vi "GOOP PROBE.vi"(11 "Probed Object":refnum<class>) -> (2 "Value String":string, 3 "Boolean":bool)   [LabVIEW 2019, in "GOOP Probe.lvlib"]
uses:
  GOOP Probe/GOOP Probe.lvlib
panel:
  out "Class Name":string
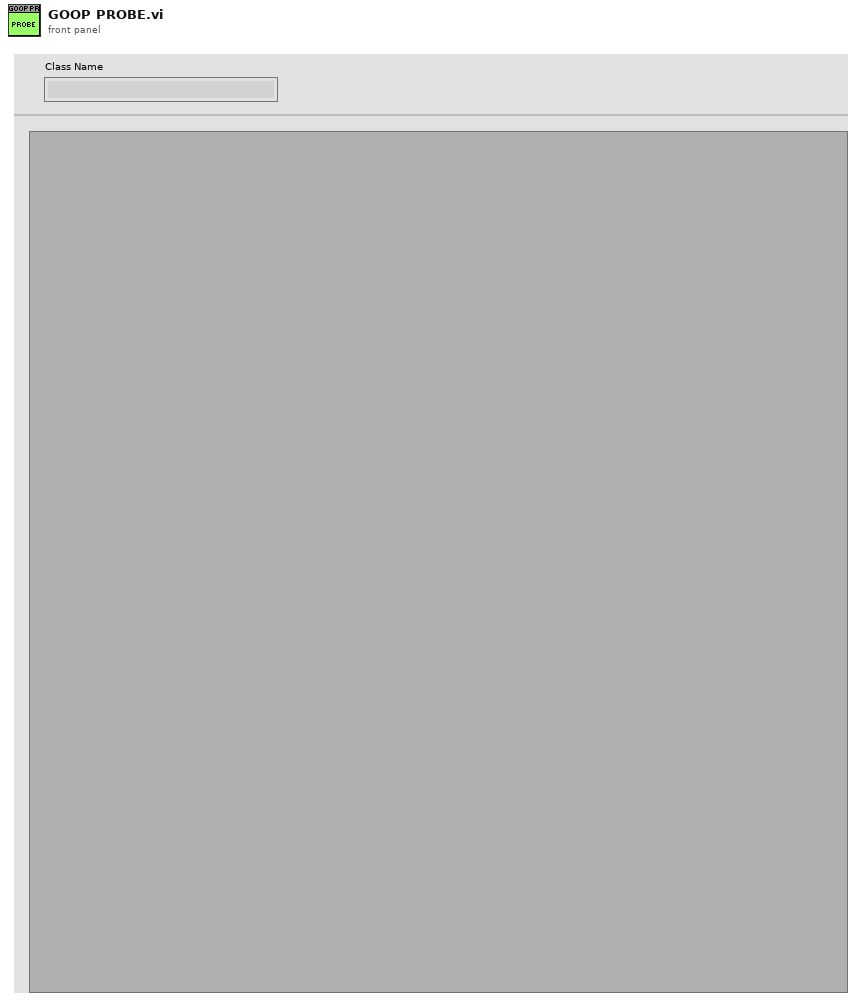
[diagram p1: front panel]
types:
  T1 = cluster{"Base Folder":path, "Cache Folder":path, "Cached Probe VI":path}
  T2 = cluster{"Object":refnum<class>, "FQN":string, "Class Name":string}
  T3 = typedef "GOOP Probe.lvlib/Level Data.ctl" = cluster{"Refnum":i32, "FQN":string, "Class Name":string, "ObjAtt.ctl Path":path, "Type":refnum<class>}
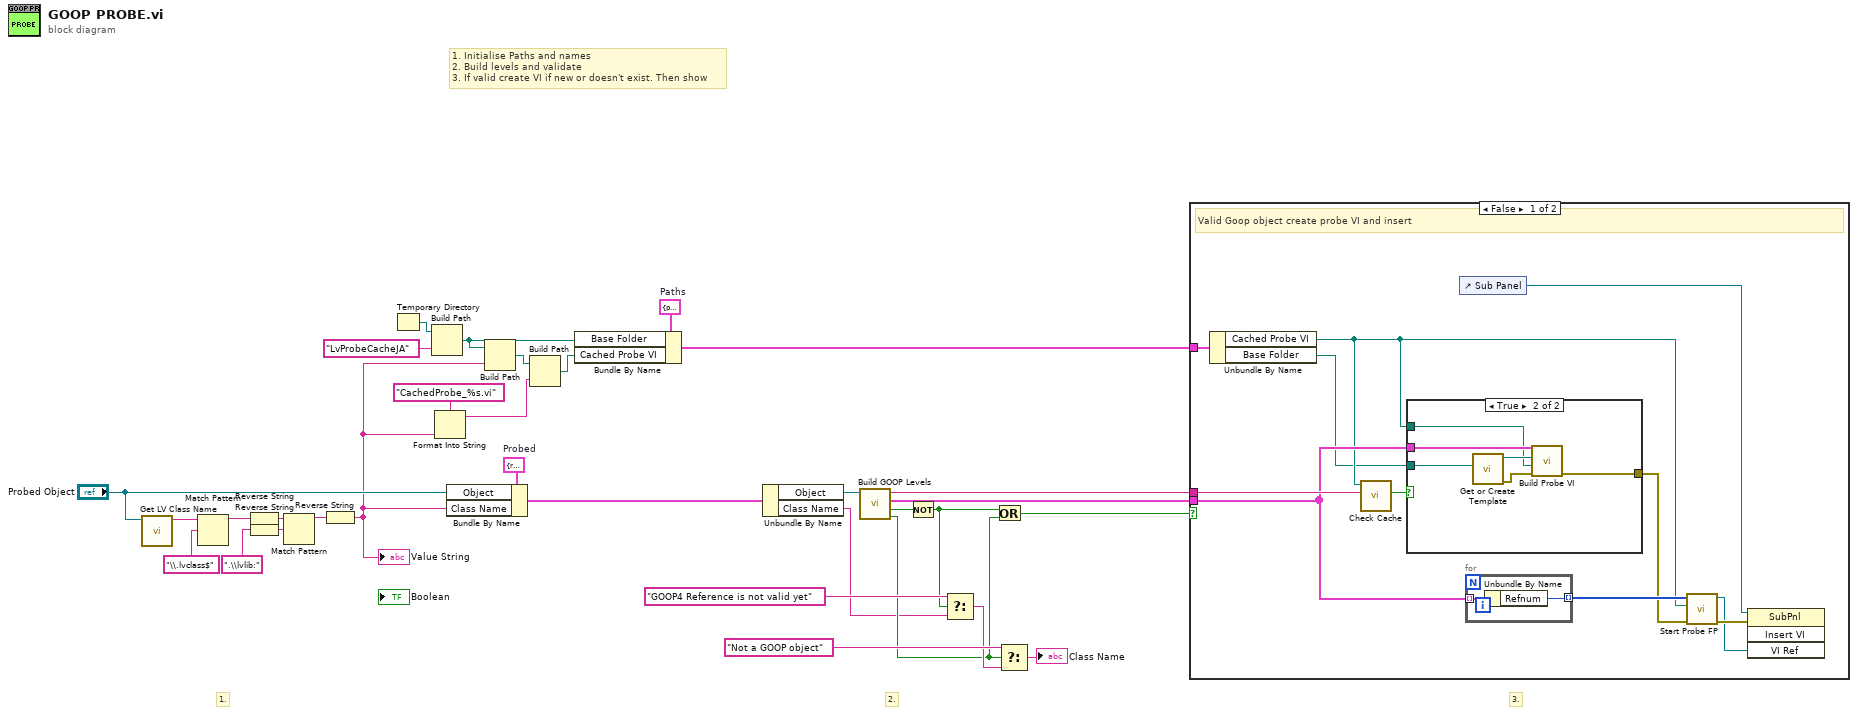
[diagram p0: block diagram]
diagram:
  w19 = T1 {"Base Folder"=path "", "Cache Folder"=path "", "Cached Probe VI"=path ""}  # Paths
  w25 = T2 {"Object"=refnum, "FQN"="", "Class Name"=""}  # Probed
  # "1. Initialise Paths and names\n2. Build levels and validate\n3. If valid create VI if new or doesn't exist. Then show"
  # "3."
  # "2."
  # "1."
  n1 = call <vilib>:"Get LV Class Name.vi"("object"="Probed Object") -> ("class name"=w31:string)  [unwired: 9 in, 1 out]
  n2 = Match Pattern(string=w31, regular expression="\\.lvclass$") -> (before substring=w30:string)  [unwired: 1 in, 3 out]
  n3 = Reverse String(1:w30) -> (0:w27:string)
  n4 = Reverse String(1:".\\lvlib:" ("regular expression")) -> (0:w28:string)
  n5 = Match Pattern(string=w27, regular expression=w28) -> (before substring=w32:string)  [unwired: 1 in, 3 out]
  n6 = Reverse String(1:w32) -> (0:w4:string)
  "Value String" <- w4
  n7 = Temporary Directory() -> (w21:path)
  n8 = Build Path(base path=w21, name or relative path="LvProbeCacheJA") -> (appended path=w18:path)
  n9 = Format Into String(format string="CachedProbe_%s.vi" ("string"), w4) -> (resulting string=w16:string)  [unwired: 2 in, 1 out]
  n10 = Bundle By Name(cluster=w25, "Object"="Probed Object", "Class Name"=w4) -> (w24:T2)
  n11 = Build Path(base path=w18, name or relative path=w4) -> (appended path=w15:path)
  n12 = Build Path(base path=w15, name or relative path=w16) -> (appended path=w14:path)
  n13 = Bundle By Name(cluster=w19, "Base Folder"=w18, "Cached Probe VI"=w14) -> (w1:T1)
  n14 = Unbundle By Name(w24) -> ("Object"=w23:refnum<class>, "Class Name"=w3:string)
  n15 = call "Build GOOP Levels.vi"("LabVIEW Object in"=w23) -> ("Not a GOOP obj?"=w6:bool, "Not a Ref Yet?"=w8:bool, "Level's Data (Child -> Parent)"=w13:T3[], "Hash"=w22:string)  [unwired: 7 in]
  n16 = Not(x=w8) -> (.not. x?=w5:bool)
  n17 = Select(t="GOOP4 Reference is not valid yet", s=w5, f=w3) -> (s? t:f=w10:string)
  n18 = Or(x=w5, y=w6) -> (x .or. y?=w2:bool)
  n19 = Select(t="Not a GOOP object", s=w6, f=w10) -> (s? t:f=→"Class Name":string)
  n20 = case shown="False" w2 {
    tunnel: w22 -> [w43 _]
    tunnel: w13 -> [w41 _]
    tunnel: w1 -> [w36 _]
    frame False {
      # "Valid Goop object create probe VI and insert"
      n21 = Unbundle By Name(w36) -> ("Cached Probe VI"=w35:path, "Base Folder"=w34:path)
      n22 = call "Check Cache.vi"("Hash"=w43, "Probe Cache Folder"=w35) -> ("Create New Probe VI?"=w42:bool)  [unwired: 9 in]
      n23 = case shown="True" w42 {
        tunnel: w35 -> [_ w46]
        tunnel: w41 -> [_ w47]
        tunnel: [_ w45] -> w37
        tunnel: w34 -> [_ w44]
        frame False {
        }
        frame True {
          n24 = call "Get or Create Template.vi"("Base Folder"=w44) -> ("error out"=w49:errorcluster, "Template Clone Ref"=w48:refnum<vi>)  [unwired: 9 in]
          n25 = call "Build Probe VI.vi"("error in"=w49, "Cache Probe VI"=w46, "VI in"=w48, "Level's Data in"=w47) -> ("error out"=w45:errorcluster)  [unwired: 7 in]
        }
      }
      n26 = control-ref of="Sub Panel"() -> (w33:refnum<vi>)
      n27 = for {
        tunnel: w41 -> [w51] mode=indexing
        tunnel: [w50] -> w40 mode=indexing
        n28 = Unbundle By Name(w51) -> ("Refnum"=w50:i32)
      }
      n29 = call "Start Probe FP.vi"("error in (no error)"=w37, "Cached Probe vi path"=w35, "Refnums"=w40) -> ("error out"=w39:errorcluster, "Probe VI"=w38:refnum<vi>)  [unwired: 7 in]
      n30 = invoke class="SubPnl" method="Insert VI"(reference=w33, error in=w39, "VI Ref"=w38) -> ()  [unwired: 1 in, 4 out]
    }
    frame True {
      # "Not a valid goop object"
    }
  }
